vi "Upload File to Database Item (File).vi"(8 "error in (no error)":errorcluster, 9 "file path":path, 10 "database item id":u32, 11 "eLab in":refnum<class "PL eLabFTW Client.lvclass">) -> (0 "error out":errorcluster, 2 "file id":u32, 3 "eLab out":refnum<class "PL eLabFTW Client.lvclass">)   [LabVIEW 2015, in "PL eLabFTW Client.lvclass"]
doc: "Uploads file to the database item and returns new file id."
uses:
  PL eLabFTW Client.lvclass
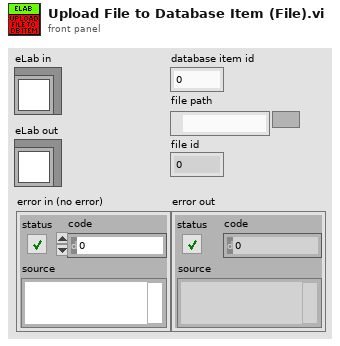
[diagram p1: front panel]
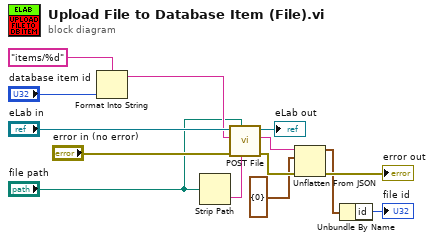
[diagram p0: block diagram]
diagram:
  n1 = Format Into String(format string="items/%d", "database item id") -> (resulting string=w10:string)  [unwired: 2 in, 1 out]
  n2 = Strip Path(path="file path") -> (name=w7:string)  [unwired: 1 out]
  n3 = call "POST File.vi"("server file name"=w7, "file path"="file path", "error in (no error)"="error in (no error)", "relative URL"=w10, "eLab in"="eLab in") -> ("error out"=w4:errorcluster, "response body"=w5:string, "eLab out"=→"eLab out":refnum<class "PL eLabFTW Client.lvclass">)  [unwired: 4 in]
  n4 = Unflatten From JSON(JSON string=w5, type and defaults=cluster{"id":u32} {"id"=0}, error in (no error)=w4) -> (value=w2:cluster{"id":u32}, error out=→"error out":errorcluster)  [unwired: 4 in]
  n5 = Unbundle By Name(w2) -> ("id"=→"file id":u32)
